vi "Write spreadsheet to file with prompt.vi"(2 "prompt":string="Choose file to write.", 4 "transpose? (no:F)":bool, 5 "delimiter (comma)":string=",", 6 "append to file? (new file:F)":bool, 7 "1D data":string[](array[string]), 8 "error in (no error)":errorcluster, 9 "2D data":string[][](array[string]), 10 "file path (dialog if empty)":path, 11 "format (%s)":string="%s") -> (0 "error out":errorcluster)   [LabVIEW 2013]
uses:
  <vilib>/Utility/error.llb/DialogType.ctl
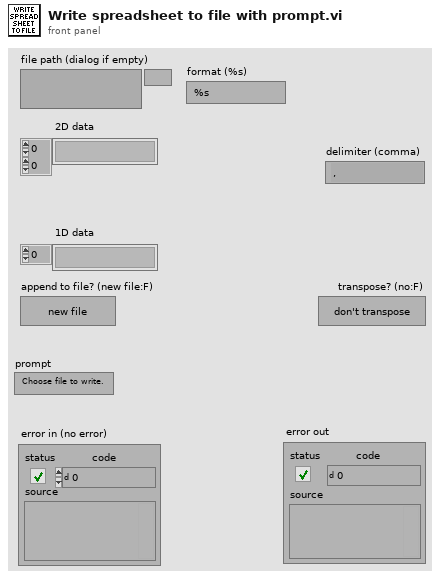
[diagram p1: front panel]
types:
  T1 = typedef "DialogType.ctl" = u16
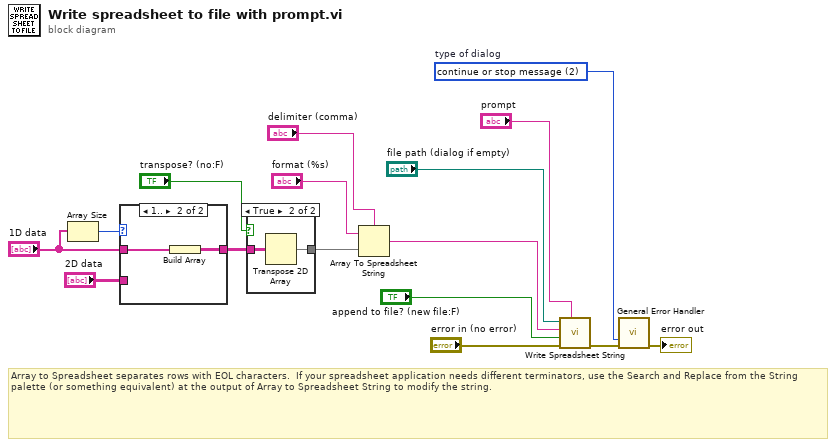
[diagram p0: block diagram]
diagram:
  w3 = T1 2 items=["no dialog", "OK message", "continue or stop message", "OK message + warnings", "continue/stop + warnings"]  # type of dialog
  # "Array to Spreadsheet separates rows with EOL characters.  If your spreadsheet application needs different terminators, use the Search and Replace from the String palette (or something equivalent) at the output of Array to Spreadsheet String to modify the string."
  n1 = Array Size(array="1D data") -> (size(s)=w16:i32)
  n2 = case shown="1.." w16 {
    tunnel: "1D data" -> [_ w19]
    tunnel: [w17 w18] -> w12
    tunnel: "2D data" -> [w17 _]
    frame ..0 {
      # "1D array is empty"
    }
    frame 1.. {
      n3 = Build Array(w19) -> (w18:string[][])
    }
  }
  n4 = case shown="True" "transpose? (no:F)" {
    tunnel: [w20 w22] -> w10
    tunnel: w12 -> [w20 w21]
    frame False {
    }
    frame True {
      n5 = Transpose 2D Array(2D array=w21) -> (transposed array=w22:string[][])
    }
  }
  n6 = Array To Spreadsheet String(delimiter (Tab)="delimiter (comma)", array=w10, 3:"format (%s)") -> (spreadsheet string=w5:string)
  n7 = call <vilib>:"Write Spreadsheet String.vi"("prompt"="prompt", "error in"="error in (no error)", "append to file? (new file:F)"="append to file? (new file:F)", "spreadsheet string"=w5, "file path (dialog if empty)"="file path (dialog if empty)") -> ("error out"=w4:errorcluster)  [unwired: 5 in, 1 out]
  n8 = call <vilib>:"General Error Handler.vi"("type of dialog (OK msg:1)"=w3, "error in (no error)"=w4) -> ("error out"=→"error out":errorcluster)  [unwired: 9 in, 4 out]
